vi "PreUUT Dialog.v2.vi"(8 "error in (no error)":errorcluster, 11 "Valid Part Numbers":string[](array[string])) -> (0 "error out":errorcluster, 1 "Comments Out":string, 2 "Part Number Out":string(combo), 3 "Cancelled?":bool, 5 "Serial Number Out":string)   [LabVIEW 2020]
doc: "Use this template to create a dialog box with event handling."
uses:
  <vilib>/regexp/Match Regular Expression.xnode
panel:
  in  "Part Number OK":bool
  in  "Serial Number OK":bool
  in  "Part Number":string(combo)
  in  "Enter UUT Serial Number":string
  in  "Cancel":bool
  in  "OK":bool
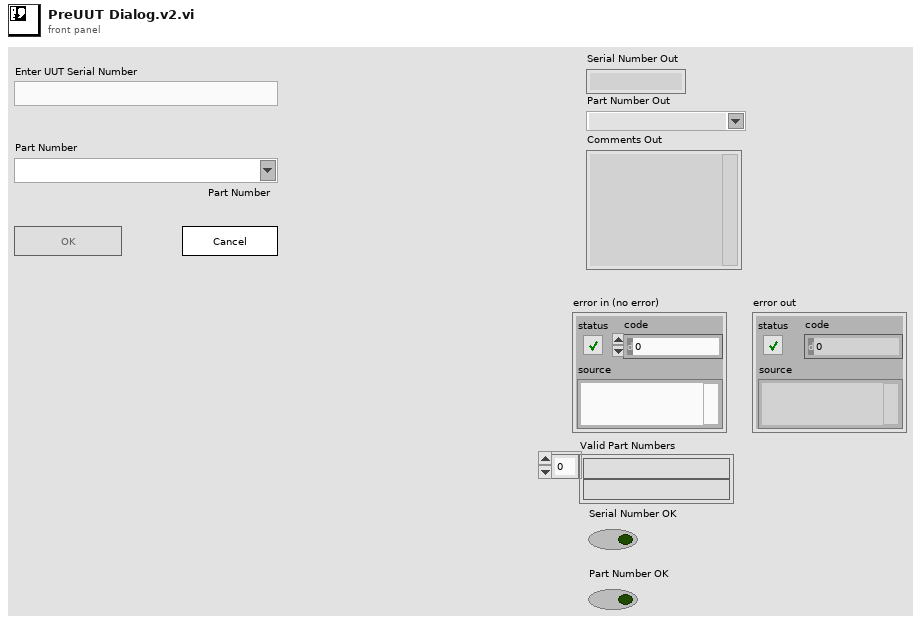
[diagram p1: front panel]
types:
  T1 = enum8{"Enabled", "Disabled", "Disabled and Grayed Out"}
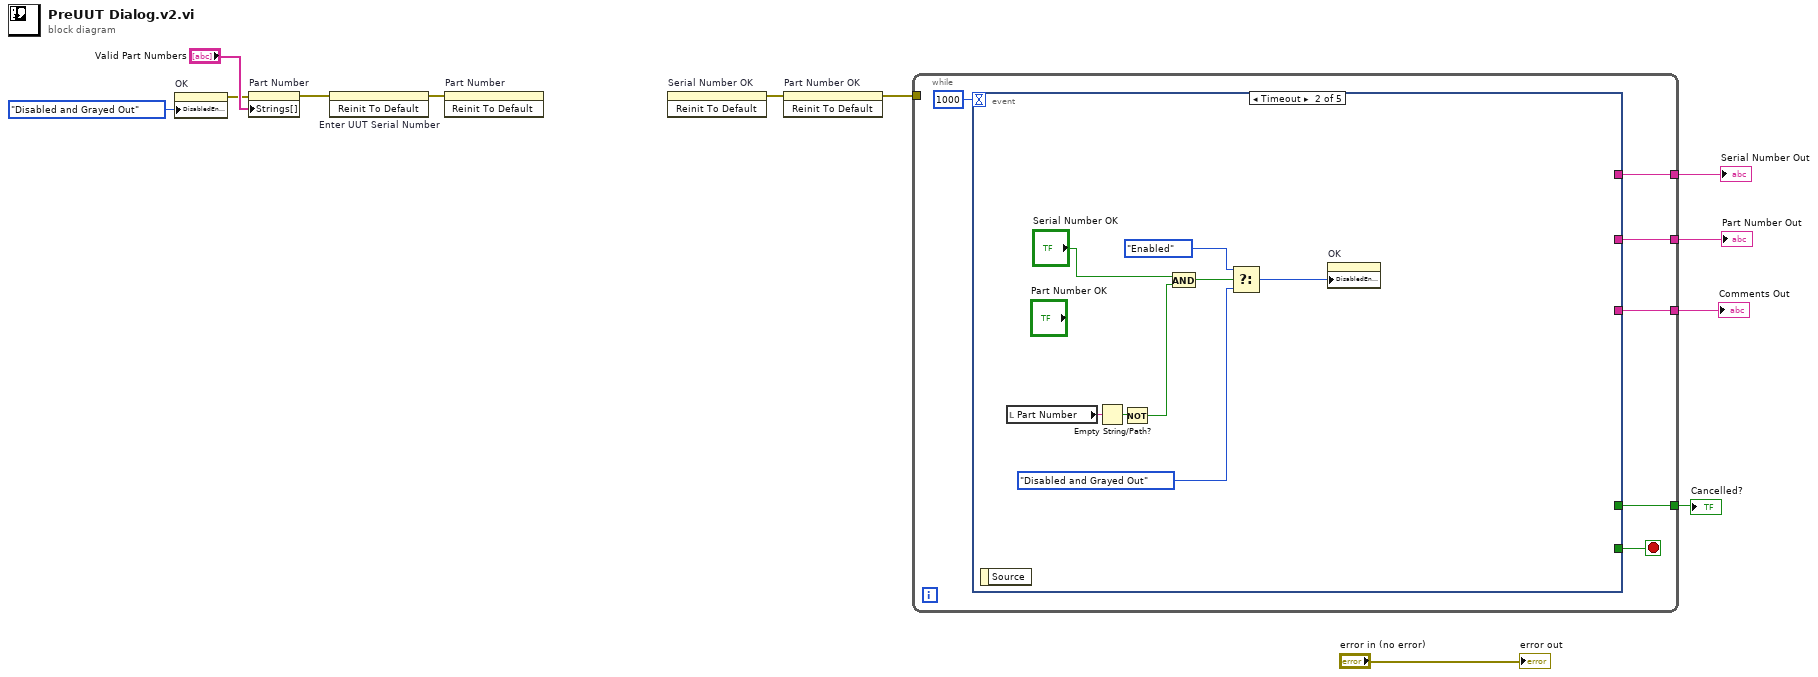
[diagram p0: block diagram]
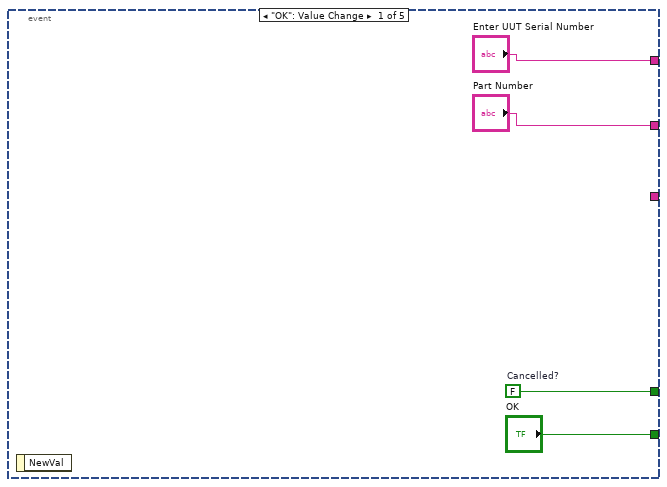
[diagram p2: hidden frame]
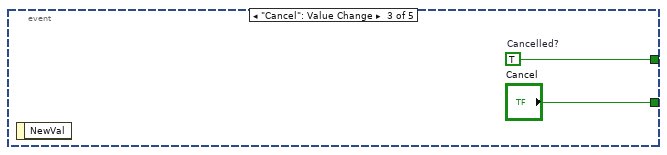
[diagram p3: hidden frame]
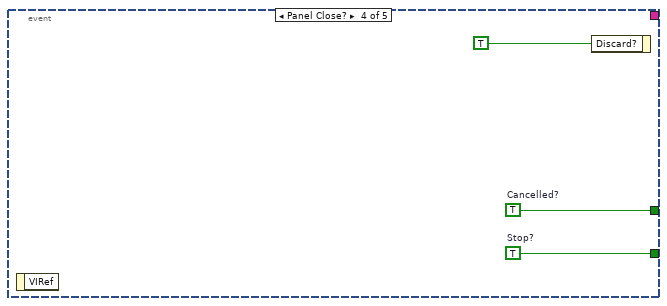
[diagram p4: hidden frame]
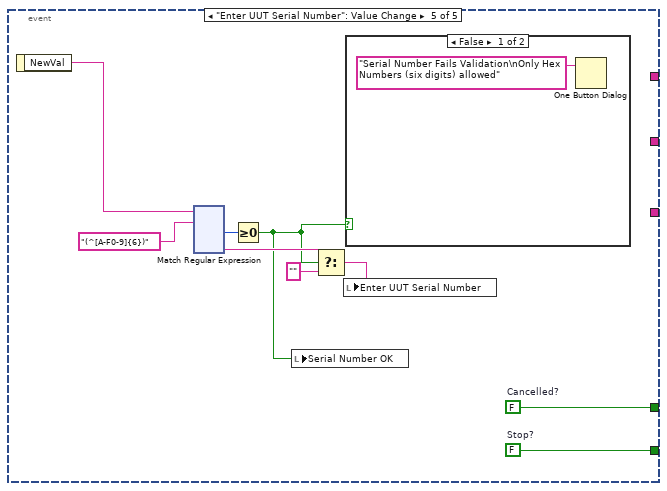
[diagram p5: hidden frame]
diagram:
  n1 = property on="OK" class="Bool"("DisabledEnum"=T1."Disabled and Grayed Out" ("Disabled")) -> (error out=w4:errorcluster)  [unwired: 2 in, 1 out]
  n2 = property on="Part Number" class="CmbBox"(error in=w4, "Strings[]"="Valid Part Numbers") -> (error out=w6:errorcluster)  [unwired: 1 in, 1 out]
  n3 = invoke on="Enter UUT Serial Number" class="Str" method="Reinit To Default"(error in=w6) -> (error out=w7:errorcluster)  [unwired: 2 in, 2 out]
  n4 = invoke on="Part Number" class="CmbBox" method="Reinit To Default"(error in=w7) -> ()  [unwired: 2 in, 3 out]
  n5 = invoke on="Serial Number OK" class="Bool (strict)" method="Reinit To Default"() -> (error out=w2:errorcluster)  [unwired: 3 in, 2 out]
  n6 = invoke on="Part Number OK" class="Bool (strict)" method="Reinit To Default"(error in=w2) -> (error out=w1:errorcluster)  [unwired: 2 in, 2 out]
  n7 = while {
    tunnel: [w17] -> w12
    tunnel: [w16] -> w11
    tunnel: [w15] -> w10
    tunnel: [w14] -> w9
    tunnel: w1 -> [_]
    stop <- w18 stop-if-true
    n8 = event shown="[1] Timeout" {
      selector: _ -> [_ _ _ _ _]
      dyn-events: _ -> [_ _ _ _ _]
      timeout: 1000 -> [_ _ _ _ _]
      tunnel: ["OK" _ "Cancel" w35 w45] -> w18
      tunnel: [w23 _ w33 w34 w44] -> w17
      tunnel: ["Enter UUT Serial Number" _ _ _ _] -> w16
      tunnel: ["Part Number" _ _ _ _] -> w15
      tunnel: [w19 _ _ _ _] -> w14
      event "OK": Value Change {
        w23 = FALSE  # Cancelled?
        n9 = event-data() -> ()  [unwired: 1 in, 1 out]
      }
      event Timeout {
        n10 = event-data() -> ()  [unwired: 1 in, 1 out]
        n11 = local read "Part Number"() -> (w26:string)
        n12 = Empty String/Path?(string/path=w26) -> (empty?=w25:bool)
        n13 = Not(x=w25) -> (.not. x?=w24:bool)
        n14 = And(x="Serial Number OK", y=w24) -> (x .and. y?=w28:bool)
        n15 = Select(t=T1."Enabled" ("Disabled"), s=w28, f=T1."Disabled and Grayed Out" ("Disabled")) -> (s? t:f=w27:T1)
        n16 = property on="OK" class="Bool"("DisabledEnum"=w27) -> ()  [unwired: 2 in, 2 out]
      }
      event "Cancel": Value Change {
        w33 = TRUE  # Cancelled?
        n17 = event-data() -> ()  [unwired: 1 in, 1 out]
      }
      event Panel Close? {
        w34 = TRUE  # Cancelled?
        w35 = TRUE  # Stop?
        n18 = event-data() -> ()  [unwired: 1 in, 1 out]
        n19 = event-data("Discard?"=TRUE) -> ()  [unwired: 1 in, 1 out]
      }
      event "Enter UUT Serial Number": Value Change {
        w44 = FALSE  # Cancelled?
        w45 = FALSE  # Stop?
        n20 = event-data() -> ("NewVal"=w42:string)  [unwired: 1 in]
        n21 = xnode "Match Regular Expression"("input string"=w42, "regular expression"="(^[A-F0-9]{6})") -> ("offset past match"=w43:i32, "submatch 1"=w40:string)  [unwired: 4 in, 4 out]
        n22 = Greater Or Equal To 0?(x=w43) -> (x >= 0?=w37:bool)
        n23 = local write "Serial Number OK"(w37) -> ()
        n24 = Select(t=w40, s=w37, f="") -> (s? t:f=w38:string)
        n25 = local write "Enter UUT Serial Number"(w38) -> ()
        n26 = case shown="False" w37 {
          frame False {
            n27 = One Button Dialog(message="Serial Number Fails Validation\nOnly Hex Numbers (six digits) allowed") -> ()  [unwired: 1 in, 1 out]
          }
          frame True {
          }
        }
      }
    }
  }
  "Cancelled?" <- w12
  "Serial Number Out" <- w11
  "Part Number Out" <- w10
  "Comments Out" <- w9
  "error out" <- "error in (no error)"
